vi "Read RP Transceiver.vi"(8 "error in (no error)":errorcluster, 11 "Red Pitaya Transceiver Driver in":refnum<class "Red Pitaya Transceiver Driver.lvclass">) -> (0 "error out":errorcluster, 2 "RP Transceiver.lvclass":refnum<class "RP Transceiver.lvclass">, 3 "Red Pitaya Transceiver Driver out":refnum<class "Red Pitaya Transceiver Driver.lvclass">)   [LabVIEW 2019, in "Red Pitaya Transceiver Driver.lvclass"]
uses:
  Red Pitaya Transceiver Driver.lvclass
  RP Transceiver/RP Transceiver.lvclass
  Red Pitaya Transceiver Driver.lvclass/Red Pitaya Transceiver Driver.ctl
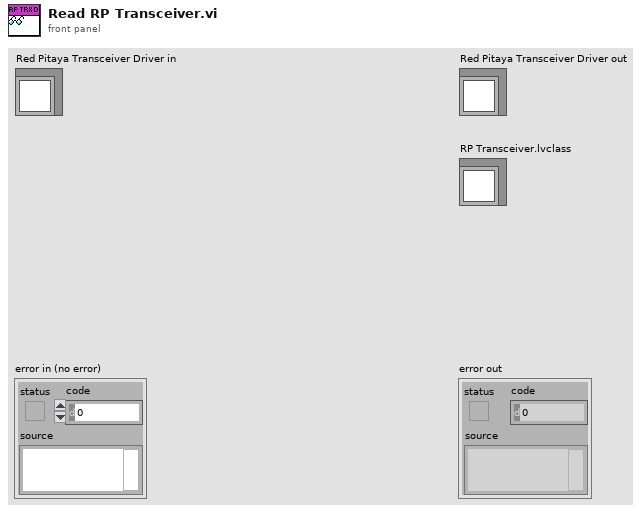
[diagram p1: front panel]
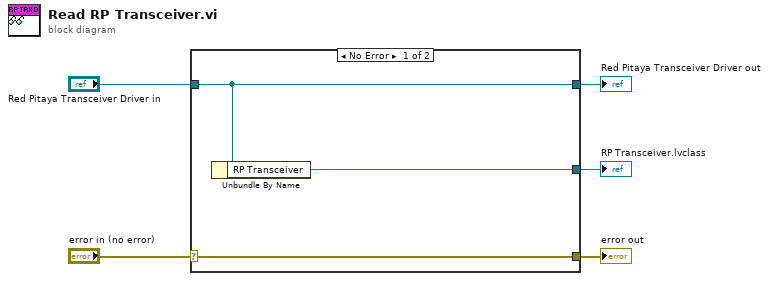
[diagram p0: block diagram]
diagram:
  n1 = case shown="No Error" "error in (no error)" {
    selector: "error in (no error)" -> [w8 w9]
    tunnel: [w8 w9] -> w4
    tunnel: [w7 w10] -> w2
    tunnel: "Red Pitaya Transceiver Driver in" -> [w7 w10]
    tunnel: [w6 _] -> w1
    frame No Error {
      n2 = Unbundle By Name(w7) -> ("RP Transceiver"=w6:refnum<class "RP Transceiver.lvclass">)
    }
    frame Error {
    }
  }
  "error out" <- w4
  "Red Pitaya Transceiver Driver out" <- w2
  "RP Transceiver.lvclass" <- w1
